vi "Snake.vi"() -> ()   [LabVIEW 2020]
uses:
  <vilib>/event_ctls.llb/eventvkey.ctl
panel:
  in  "stop 2":bool
  in  "Wybierz poziom trudności":u16(ring) items=["B. Trudny", "trudny", "średni", "łatwy"]
  in  "stop":bool
  out "Array 5":u32[][](array[colorbox])
  out "punkty":i32
  in  "Start":bool
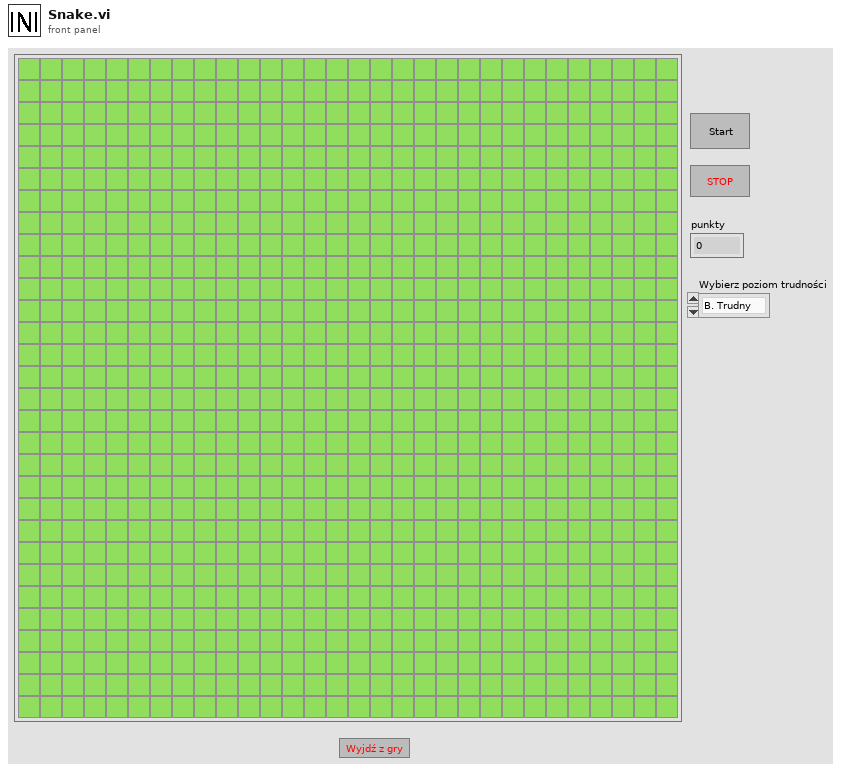
[diagram p1: front panel]
types:
  T1 = enum8{"Enabled", "Disabled", "Disabled and Grayed Out"}
  T2 = typedef "eventvkey.ctl" = enum16{"ASCII", "Enter", "Return", "Shift", "Ctrl", "Alt", "Cmd", "Opt", "Caps", "NumLock", "Clear", "Break", "Up", "Down", "Left", "Right", "Insert", "Delete", "Home", "End", "PageUp", "PageDown", "Escape", "Help", "Pause", "ScrollLock", "F1", "F2", "F3", "F4", "F5", "F6", "F7", "F8", "F9", "F10", "F11", "F12", "F13", "F14", "F15", "F16", "F17", "F18", "F19", "F20", "F21", "F22", "F23", "F24", "Play", "VolumeUp", "VolumeDown", "Mute", "Two Byte Char"}
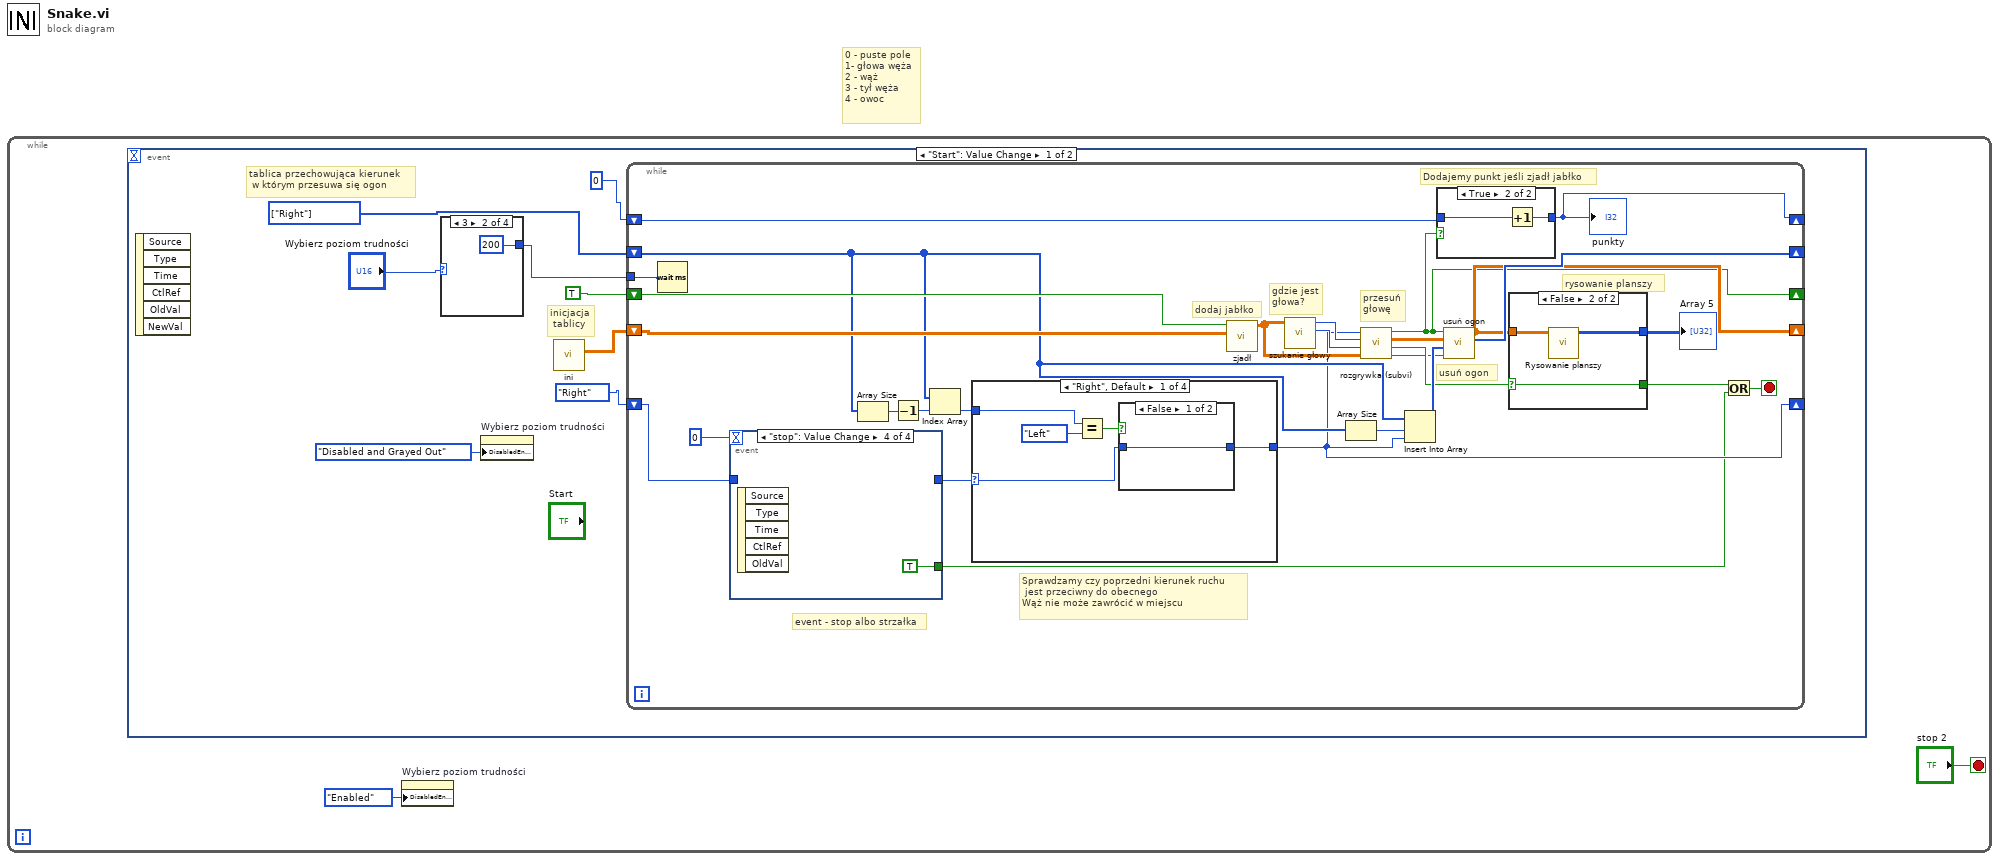
[diagram p0: block diagram]
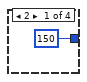
[diagram p2: hidden frame]
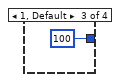
[diagram p3: hidden frame]
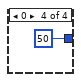
[diagram p4: hidden frame]
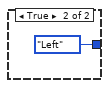
[diagram p6: hidden frame]
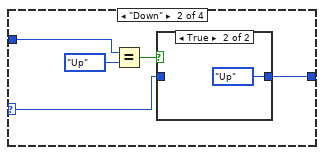
[diagram p7: hidden frame]
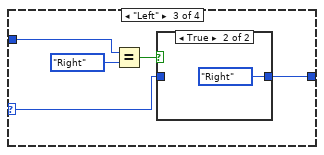
[diagram p9: hidden frame]
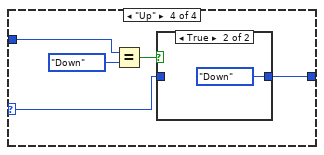
[diagram p11: hidden frame]
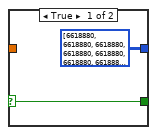
[diagram p13: hidden frame]
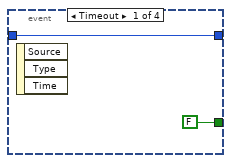
[diagram p14: hidden frame]
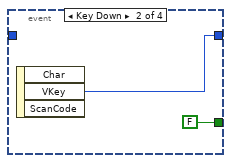
[diagram p15: hidden frame]
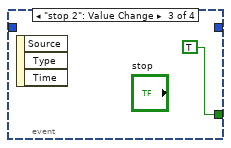
[diagram p16: hidden frame]
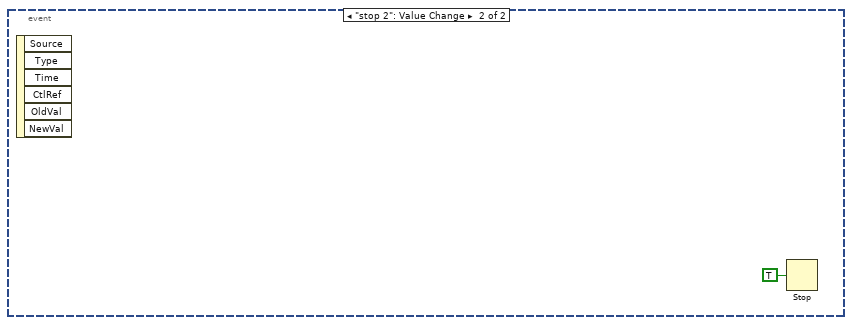
[diagram p17: hidden frame]
diagram:
  # "0 - puste pole\n1- głowa węża\n2 - wąż\n3 - tył węża\n4 - owoc"
  n1 = while {
    stop <- "stop 2" stop-if-true
    n2 = event shown="[0] \"Start\": Value Change" {
      selector: _ -> [_ _]
      dyn-events: _ -> [_ _]
      timeout: _ -> [_ _]
      event "Start": Value Change {
        w8 = T2[] [enum."Right"] items=["ASCII", "Enter", "Return", "Shift", "Ctrl", "Alt", "Cmd", "Opt", "Caps", "NumLock", "Clear", "Break", "Up", "Down", "Left", "Right", "Insert", "Delete", "Home", "End", "PageUp", "PageDown", "Escape", "Help", "Pause", "ScrollLock", "F1", "F2", "F3", "F4", "F5", "F6", "F7", "F8", "F9", "F10", "F11", "F12", "F13", "F14", "F15", "F16", "F17", "F18", "F19", "F20", "F21", "F22", "F23", "F24", "Play", "VolumeUp", "VolumeDown", "Mute", "Two Byte Char"] ("array")
        # "tablica przechowująca kierunek\n w którym przesuwa się ogon"
        # "inicjacja\n tablicy"
        n3 = event-data() -> ()  [unwired: 1 in, 6 out]
        n4 = case shown="3" "Wybierz poziom trudności" {
          tunnel: [150 200 100 50] -> w6
          frame 2 {
          }
          frame 3 {
          }
          frame 1, Default {
          }
          frame 0 {
          }
        }
        n5 = property on="Wybierz poziom trudności" class="Ring (strict)"("DisabledEnum"=T1."Disabled and Grayed Out" ("Disabled")) -> ()  [unwired: 2 in, 2 out]
        n6 = call "ini.vi"() -> ("Array 2"=w5:dbl[][])  [unwired: 11 in]
        n7 = while {
          shift-right: [w33] -> _
          shift-left: w5 -> [w31]
          shift-right: [w24] -> _
          shift-left: eventvkey."Right" ("Obecny ruch") -> [w40]
          shift-right: [w38] -> _
          shift-left: w8 -> [w29]
          shift-right: [w23] -> _
          shift-left: TRUE -> [w32]
          shift-right: [w21] -> _
          shift-left: 0 -> [w22]
          tunnel: w6 -> [w19]
          stop <- w16 stop-if-true
          # "dodaj jabłko"
          # "Dodajemy punkt jeśli zjadł jabłko"
          # "Sprawdzamy czy poprzedni kierunek ruchu\n jest przeciwny do obecnego\nWąż nie może zawrócić w miejscu"
          # "event - stop albo strzałka"
          # "usuń ogon"
          # "przesuń\ngłowę"
          # "gdzie jest\ngłowa?"
          # "rysowanie planszy"
          n8 = Wait (ms)(milliseconds to wait=w19) -> ()  [unwired: 1 out]
          n9 = event shown="[3] \"stop\": Value Change" {
            selector: _ -> [_ _ _ _]
            dyn-events: _ -> [_ _ _ _]
            timeout: 0 -> [_ _ _ _]
            tunnel: [w80 w82 _ _] -> w26
            tunnel: w40 -> [w80 _ _ _]
            tunnel: [FALSE ("stop") FALSE ("stop") TRUE ("stop") TRUE ("stop")] -> w15
            event Timeout {
              n10 = event-data() -> ()  [unwired: 1 in, 3 out]
            }
            event Key Down {
              n11 = event-data() -> ("VKey"=w82:T2)  [unwired: 1 in, 2 out]
            }
            event "stop 2": Value Change {
              n12 = event-data() -> ()  [unwired: 1 in, 3 out]
            }
            event "stop": Value Change {
              n13 = event-data() -> ()  [unwired: 1 in, 5 out]
            }
          }
          n14 = Array Size(array=w29) -> (size(s)=w28:i32)
          n15 = Decrement(x=w28) -> (x-1=w27:i32)
          n16 = Index Array(array=w29, index=w27) -> (element=w25:T2)
          n17 = case shown="\"Right\", Default" w26 {
            selector: w26 -> [w46 w53 w60 w67]
            tunnel: w25 -> [w50 w57 w64 w71]
            tunnel: [w47 w54 w61 w68] -> w24
            frame "Right", Default {
              n18 = Equal?(x=w50, y=eventvkey."Left" ("new element/subarray")) -> (x = y?=w48:bool)
              n19 = case shown="False" w48 {
                tunnel: [w51 eventvkey."Left" ("new element/subarray")] -> w47
                tunnel: w46 -> [w51 _]
                frame False {
                }
                frame True {
                }
              }
            }
            frame "Down" {
              n20 = Equal?(x=w57, y=eventvkey."Up" ("new element/subarray")) -> (x = y?=w55:bool)
              n21 = case shown="True" w55 {
                tunnel: [w58 eventvkey."Up" ("new element/subarray")] -> w54
                tunnel: w53 -> [w58 _]
                frame False {
                }
                frame True {
                }
              }
            }
            frame "Left" {
              n22 = Equal?(x=w64, y=eventvkey."Right" ("new element/subarray")) -> (x = y?=w62:bool)
              n23 = case shown="True" w62 {
                tunnel: [w65 eventvkey."Right" ("new element/subarray")] -> w61
                tunnel: w60 -> [w65 _]
                frame False {
                }
                frame True {
                }
              }
            }
            frame "Up" {
              n24 = Equal?(x=w71, y=eventvkey."Down" ("new element/subarray")) -> (x = y?=w69:bool)
              n25 = case shown="True" w69 {
                tunnel: [w72 eventvkey."Down" ("new element/subarray")] -> w68
                tunnel: w67 -> [w72 _]
                frame False {
                }
                frame True {
                }
              }
            }
          }
          n26 = call "zjadł.vi"("Array 2"=w31, "zjadł?"=w32) -> ("Array 3"=w30:dbl[][])  [unwired: 9 in]
          n27 = call "szukanie głowy.vi"("Array in"=w30) -> ("wiersz"=w41:i32, "kolumna"=w42:i32)  [unwired: 9 in]
          n28 = Array Size(array=w29) -> (size(s)=w37:i32)
          n29 = call "rozgrywka (subvi).vi"("Array"=w30, "wiersz"=w41, "kolumna"=w42, "VKey"=w24) -> ("Po ogonie"=w20:bool, "przegrana?"=w35:bool, "Array 2"=w34:dbl[][], "zjadł?"=w23:bool)  [unwired: 4 in]
          n30 = Insert Into Array(array=w29, index=w37, new element=w24) -> (w39:T2[])
          n31 = case shown="True" w23 {
            tunnel: w22 -> [w43 w45]
            tunnel: [w43 w44] -> w21
            frame False {
            }
            frame True {
              n32 = Increment(x=w45) -> (x+1=w44:i32)
            }
          }
          "punkty" <- w21
          n33 = call "usuń ogon.vi"("Po ogonie?"=w20, "ogon"=w39, "Array 3"=w34, "zjadł?"=w23) -> ("ogon"=w38:T2[], "Array 2"=w33:dbl[][])  [unwired: 6 in]
          n34 = case shown="False" w35 {
            selector: w35 -> [w75 w76]
            tunnel: w33 -> [_ w78]
            tunnel: [u32[][] [[6618880, 6618880, 6618880, 6618880, 6618880, 6618880, 6618880, 6618880, 6618880, 6618880, 6618880, 6618880, 6618880, 6618880, 6618880, 6618880, 6618880, 6618880, 6618880, 6618880, 6618880, 6618880, 6618880, 6618880, 6618880, 6618880, 6618880, 6618880, 6618880, 6618880, 6618880], [6618880, 6618880, 6618880, 6618880, 6618880, 6618880, 6618880, 6618880, 6618880, 6618880, 6618880, 6618880, 6618880, 6618880, 6618880, 6618880, 6618880, 6618880, 6618880, 6618880, 6618880, 6618880, 6618880, 6618880, 6618880, 6618880, 6618880, 6618880, 6618880, 6618880, 6618880], [6618880, 6618880, 6618880, 6618880, 6618880, 6618880, 6618880, 6618880, 6618880, 6618880, 6618880, 6618880, 6618880, 6618880, 6618880, 6618880, 6618880, 6618880, 6618880, 6618880, 6618880, 6618880, 6618880, 6618880, 6618880, 6618880, 6618880, 6618880, 6618880, 6618880, 6618880], [6618880, 6618880, 6618880, 6618880, 6618880, 6618880, 6618880, 0, 6618880, 6618880, 6618880, 0, 6618880, 6618880, 0, 65793, 6618880, 6618880, 0, 6618880, 6618880, 0, 6618880, 6618880, 6618880, 6618880, 6618880, 6618880, 6618880, 6618880, 6618880], [6618880, 6618880, 6618880, 6618880, 6618880, 6618880, 6618880, 0, 6618880, 6618880, 6618880, 0, 6618880, 0, 6618880, 6618880, 0, 6618880, 65793, 6618880, 6618880, 0, 6618880, 6618880, 6618880, 6618880, 6618880, 6618880, 6618880, 6618880, 6618880], [6618880, 6618880, 6618880, 6618880, 6618880, 6618880, 6618880, 0, 6618880, 6618880, 6618880, 0, 6618880, 0, 6618880, 6618880, 0, 6618880, 0, 6618880, 6618880, 0, 6618880, 6618880, 6618880, 6618880, 6618880, 6618880, 6618880, 6618880, 6618880], [6618880, 6618880, 6618880, 6618880, 6618880, 6618880, 6618880, 6618880, 0, 6618880, 0, 6618880, 6618880, 0, 6618880, 6618880, 0, 6618880, 0, 6618880, 6618880, 0, 6618880, 6618880, 6618880, 6618880, 6618880, 6618880, 6618880, 6618880, 6618880], [6618880, 6618880, 6618880, 6618880, 6618880, 6618880, 6618880, 6618880, 6618880, 0, 6618880, 6618880, 6618880, 0, 6618880, 6618880, 0, 6618880, 0, 6618880, 6618880, 0, 6618880, 6618880, 6618880, 6618880, 6618880, 6618880, 6618880, 6618880, 6618880], [6618880, 6618880, 6618880, 6618880, 6618880, 6618880, 6618880, 6618880, 6618880, 0, 6618880, 6618880, 6618880, 0, 6618880, 6618880, 0, 6618880, 0, 6618880, 6618880, 0, 6618880, 6618880, 6618880, 6618880, 6618880, 6618880, 6618880, 6618880, 6618880], [6618880, 6618880, 6618880, 6618880, 6618880, 6618880, 6618880, 6618880, 6618880, 0, 6618880, 6618880, 6618880, 6618880, 0, 0, 6618880, 6618880, 6618880, 0, 0, 6618880, 6618880, 6618880, 6618880, 6618880, 6618880, 6618880, 6618880, 6618880, 6618880], [6618880, 6618880, 6618880, 6618880, 6618880, 6618880, 6618880, 6618880, 6618880, 6618880, 6618880, 6618880, 6618880, 6618880, 6618880, 6618880, 6618880, 6618880, 6618880, 6618880, 6618880, 6618880, 6618880, 6618880, 6618880, 6618880, 6618880, 6618880, 6618880, 6618880, 6618880], [6618880, 6618880, 6618880, 6618880, 6618880, 0, 6618880, 6618880, 6618880, 6618880, 6618880, 0, 0, 6618880, 6618880, 6618880, 0, 0, 6618880, 6618880, 0, 0, 0, 0, 6618880, 6618880, 6618880, 6618880, 6618880, 6618880, 6618880], [6618880, 6618880, 6618880, 6618880, 6618880, 0, 6618880, 6618880, 6618880, 6618880, 0, 6618880, 6618880, 0, 6618880, 131586, 6618880, 6618880, 0, 6618880, 0, 6618880, 6618880, 6618880, 6618880, 6618880, 6618880, 6618880, 6618880, 6618880, 6618880], [6618880, 6618880, 6618880, 6618880, 6618880, 0, 6618880, 6618880, 6618880, 6618880, 0, 6618880, 6618880, 0, 6618880, 0, 6618880, 6618880, 6618880, 6618880, 0, 6618880, 6618880, 6618880, 6618880, 6618880, 6618880, 6618880, 6618880, 6618880, 6618880], [6618880, 6618880, 6618880, 6618880, 6618880, 0, 6618880, 6618880, 6618880, 6618880, 0, 6618880, 6618880, 0, 6618880, 6618880, 0, 0, 6618880, 6618880, 131586, 0, 0, 0, 6618880, 6618880, 6618880, 6618880, 6618880, 6618880, 6618880], [6618880, 6618880, 6618880, 6618880, 6618880, 0, 6618880, 6618880, 6618880, 6618880, 0, 6618880, 6618880, 0, 6618880, 6618880, 6618880, 6618880, 0, 6618880, 0, 6618880, 6618880, 6618880, 6618880, 6618880, 6618880, 6618880, 6618880, 6618880, 6618880], [6618880, 6618880, 6618880, 6618880, 6618880, 0, 6618880, 6618880, 6618880, 6618880, 65793, 6618880, 6618880, 0, 6618880, 0, 6618880, 6618880, 0, 6618880, 0, 6618880, 6618880, 6618880, 6618880, 6618880, 6618880, 6618880, 6618880, 6618880, 6618880], [6618880, 6618880, 6618880, 6618880, 6618880, 0, 0, 0, 0, 6618880, 6618880, 0, 0, 6618880, 6618880, 6618880, 0, 0, 6618880, 6618880, 0, 0, 0, 0, 6618880, 6618880, 6618880, 6618880, 6618880, 6618880, 6618880], [6618880, 6618880, 6618880, 6618880, 6618880, 6618880, 6618880, 6618880, 6618880, 6618880, 6618880, 6618880, 6618880, 6618880, 6618880, 6618880, 6618880, 6618880, 6618880, 6618880, 6618880, 6618880, 6618880, 6618880, 6618880, 6618880, 6618880, 6618880, 6618880, 6618880, 6618880], [6618880, 6618880, 6618880, 6618880, 6618880, 6618880, 6618880, 6618880, 6618880, 6618880, 6618880, 6618880, 6618880, 6618880, 6618880, 6618880, 6618880, 6618880, 6618880, 6618880, 6618880, 6618880, 6618880, 6618880, 6618880, 6618880, 6618880, 6618880, 6618880, 6618880, 6618880], [6618880, 6618880, 6618880, 6618880, 6618880, 6618880, 6618880, 6618880, 6618880, 6618880, 6618880, 6618880, 6618880, 6618880, 6618880, 6618880, 6618880, 6618880, 6618880, 6618880, 6618880, 6618880, 6618880, 6618880, 6618880, 6618880, 6618880, 6618880, 6618880, 6618880, 6618880], [6618880, 6618880, 6618880, 6618880, 6618880, 6618880, 6618880, 6618880, 6618880, 6618880, 6618880, 6618880, 6618880, 6618880, 6618880, 6618880, 6618880, 6618880, 6618880, 6618880, 6618880, 6618880, 6618880, 6618880, 6618880, 6618880, 6618880, 6618880, 6618880, 6618880, 6618880], [6618880, 6618880, 6618880, 6618880, 6618880, 6618880, 6618880, 6618880, 6618880, 6618880, 6618880, 6618880, 6618880, 6618880, 6618880, 6618880, 6618880, 6618880, 6618880, 6618880, 6618880, 6618880, 6618880, 6618880, 6618880, 6618880, 6618880, 6618880, 6618880, 6618880, 6618880], [6618880, 6618880, 6618880, 6618880, 6618880, 6618880, 6618880, 6618880, 6618880, 6618880, 6618880, 6618880, 6618880, 6618880, 6618880, 6618880, 6618880, 6618880, 6618880, 6618880, 6618880, 6618880, 6618880, 6618880, 6618880, 6618880, 6618880, 6618880, 6618880, 6618880, 6618880], [6618880, 6618880, 6618880, 6618880, 6618880, 6618880, 6618880, 6618880, 6618880, 6618880, 6618880, 6618880, 6618880, 6618880, 6618880, 6618880, 6618880, 6618880, 6618880, 6618880, 6618880, 6618880, 6618880, 6618880, 6618880, 6618880, 6618880, 6618880, 6618880, 6618880, 6618880], [6618880, 6618880, 6618880, 6618880, 6618880, 6618880, 6618880, 6618880, 6618880, 6618880, 6618880, 6618880, 6618880, 6618880, 6618880, 6618880, 6618880, 6618880, 6618880, 6618880, 6618880, 6618880, 6618880, 6618880, 6618880, 6618880, 6618880, 6618880, 6618880, 6618880, 6618880], [6618880, 6618880, 6618880, 6618880, 6618880, 6618880, 6618880, 6618880, 6618880, 6618880, 6618880, 6618880, 6618880, 6618880, 6618880, 6618880, 6618880, 6618880, 6618880, 6618880, 6618880, 6618880, 6618880, 6618880, 6618880, 6618880, 6618880, 6618880, 6618880, 6618880, 6618880], [6618880, 6618880, 6618880, 6618880, 6618880, 6618880, 6618880, 6618880, 6618880, 6618880, 6618880, 6618880, 6618880, 6618880, 6618880, 6618880, 6618880, 6618880, 6618880, 6618880, 6618880, 6618880, 6618880, 6618880, 6618880, 6618880, 6618880, 6618880, 6618880, 6618880, 6618880], [6618880, 6618880, 6618880, 6618880, 6618880, 6618880, 6618880, 6618880, 6618880, 6618880, 6618880, 6618880, 6618880, 6618880, 6618880, 6618880, 6618880, 6618880, 6618880, 6618880, 6618880, 6618880, 6618880, 6618880, 6618880, 6618880, 6618880, 6618880, 6618880, 6618880, 6618880], [6618880, 6618880, 6618880, 6618880, 6618880, 6618880, 6618880, 6618880, 6618880, 6618880, 6618880, 6618880, 6618880, 6618880, 6618880, 6618880, 6618880, 6618880, 6618880, 6618880, 6618880, 6618880, 6618880, 6618880, 6618880, 6618880, 6618880, 6618880, 6618880, 6618880, 6618880], [6618880, 6618880, 6618880, 6618880, 6618880, 6618880, 6618880, 6618880, 6618880, 6618880, 6618880, 6618880, 6618880, 6618880, 6618880, 6618880, 6618880, 6618880, 6618880, 6618880, 6618880, 6618880, 6618880, 6618880, 6618880, 6618880, 6618880, 6618880, 6618880, 6618880, 6618880]] ("Array out") w77] -> w18
            tunnel: [w75 w76] -> w17
            frame True {
            }
            frame False {
              n35 = call "Rysowanie planszy.vi"("Array in"=w78) -> ("Array out"=w77:u32[][])  [unwired: 10 in]
            }
          }
          "Array 5" <- w18
          n36 = Or(x=w17, y=w15) -> (x .or. y?=w16:bool)
        }
      }
      event "stop 2": Value Change {
        n37 = event-data() -> ()  [unwired: 1 in, 6 out]
        n38 = Stop(stop? (T)=TRUE) -> ()
      }
    }
    n39 = property on="Wybierz poziom trudności" class="Ring (strict)"("DisabledEnum"=T1."Enabled" ("Disabled")) -> ()  [unwired: 2 in, 2 out]
  }
